vi "main.vi"() -> ()   [LabVIEW 2020]
panel:
  in  "Sun_y":dbl
  in  "Sun_x":dbl
  in  "Earth_y":dbl
  in  "Earth_x":dbl
  out "XY Graph":cluster{"Earth_x":dbl, "Earth_y":dbl}[](graph)
  in  "Stop":bool
  out "Earth Current":cluster{"Earth_x":dbl, "Earth_y":dbl}
  # "Equation of Newtonian Gravity\nF = G*(m1*m2)/r^2\n\nF=m*a\nint(int(F)) = m*s\n    ,where s = position\n                G = 6.674e-11 m^3*kg^-1*s*-2"
  # "1. How to simulate a 1D linear gravity? \nStep 0, simulate movement of a dot..."
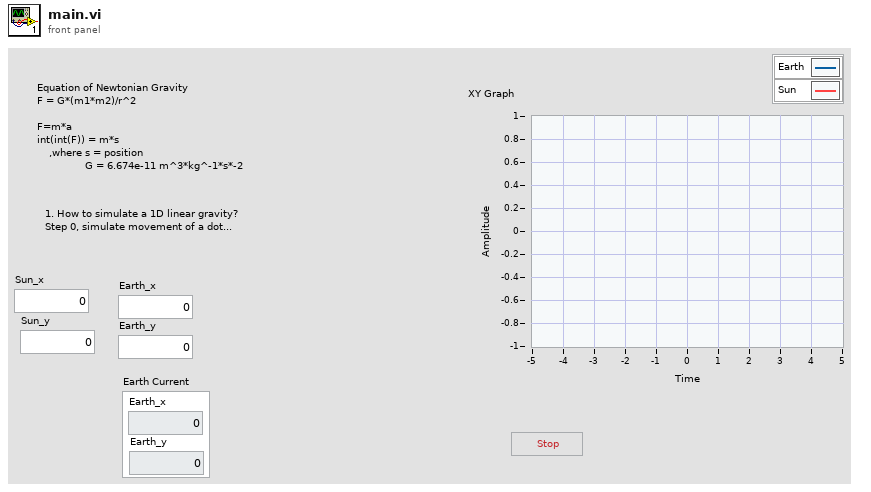
[diagram p1: front panel]
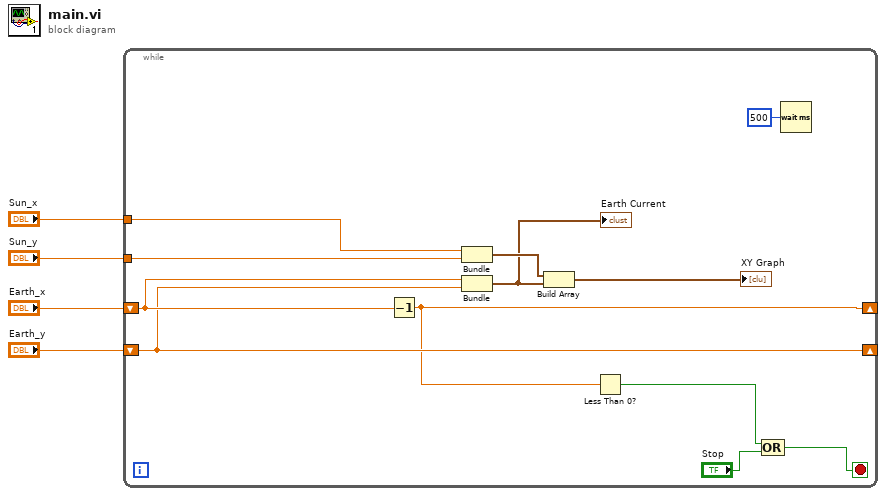
[diagram p0: block diagram]
diagram:
  n1 = while {
    tunnel: "Sun_x" -> [w16]
    tunnel: "Sun_y" -> [w15]
    shift-right: [w9] -> _
    shift-left: "Earth_x" -> [w11]
    shift-right: [w10] -> _
    shift-left: "Earth_y" -> [w10]
    stop <- w6 stop-if-true
    n2 = Decrement(x=w11) -> (x-1=w9:dbl)
    n3 = Bundle("Sun_x"=w16, "Sun_y"=w15) -> (w14:cluster{"Sun_x":dbl, "Sun_y":dbl})  [unwired: 1 in]
    n4 = Bundle("Earth_x"=w11, "Earth_y"=w10) -> (w12:cluster{"Earth_x":dbl, "Earth_y":dbl})  [unwired: 1 in]
    "Earth Current" <- w12
    n5 = Build Array(w14, w12) -> (→"XY Graph":cluster{"Earth_x":dbl, "Earth_y":dbl}[])
    n6 = Less Than 0?(x=w9) -> (x < 0?=w7:bool)
    n7 = Compound Arithmetic op=OR(w7, "Stop") -> (w6:bool)
    n8 = Wait (ms)(milliseconds to wait=u32 500) -> ()  [unwired: 1 out]
  }
